vi "Setup.vi"(0 "Scalar Path in":refnum<class "Scalar Path.lvclass">, 11 "error in (no error)":errorcluster) -> (4 "Scalar Path out":refnum<class "Scalar Path.lvclass">, 15 "error out":errorcluster)   [LabVIEW 2023, in "RFFixtureCharact.Public.lvlib" / "Scalar Path.lvclass"]
uses:
  Scalar Path.lvclass
  Common/Base Classes/Path/Path.lvclass
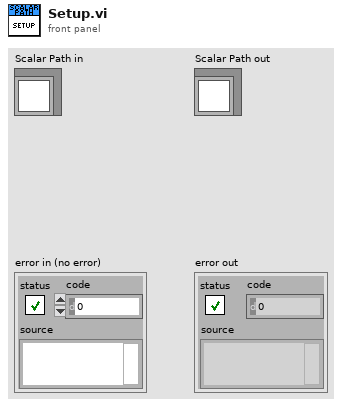
[diagram p1: front panel]
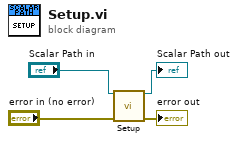
[diagram p0: block diagram]
diagram:
  n1 = call-parent "Setup.vi"("Path in"="Scalar Path in", "error in (no error)"="error in (no error)") -> ("Path out"=→"Scalar Path out":refnum<class "Scalar Path.lvclass">, "error out"=→"error out":errorcluster)  [unwired: 12 in]
